vi "Launch VI Tester.vi"(8 "error in (no error)":errorcluster, 11 "application reference":refnum<vi>) -> (0 "error out":errorcluster, 2 "Opened UI?":bool, 3 "VI Tester Ref":refnum<vi>)   [LabVIEW 2011, in "VI Tester Project API.lvlib"]
uses:
  VI Tester Project API.lvlib
panel:
  out "Status":string
  out "Version":string
  # "© 2007 - 2014 JKI. All Rights Reserved."
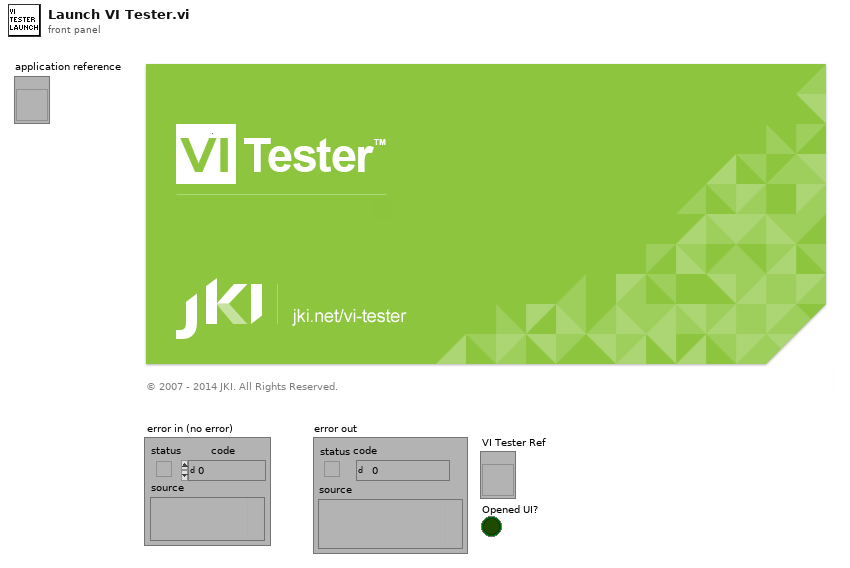
[diagram p1: front panel]
types:
  T1 = enum32{"Bad", "Idle", "Run top level", "Running"}
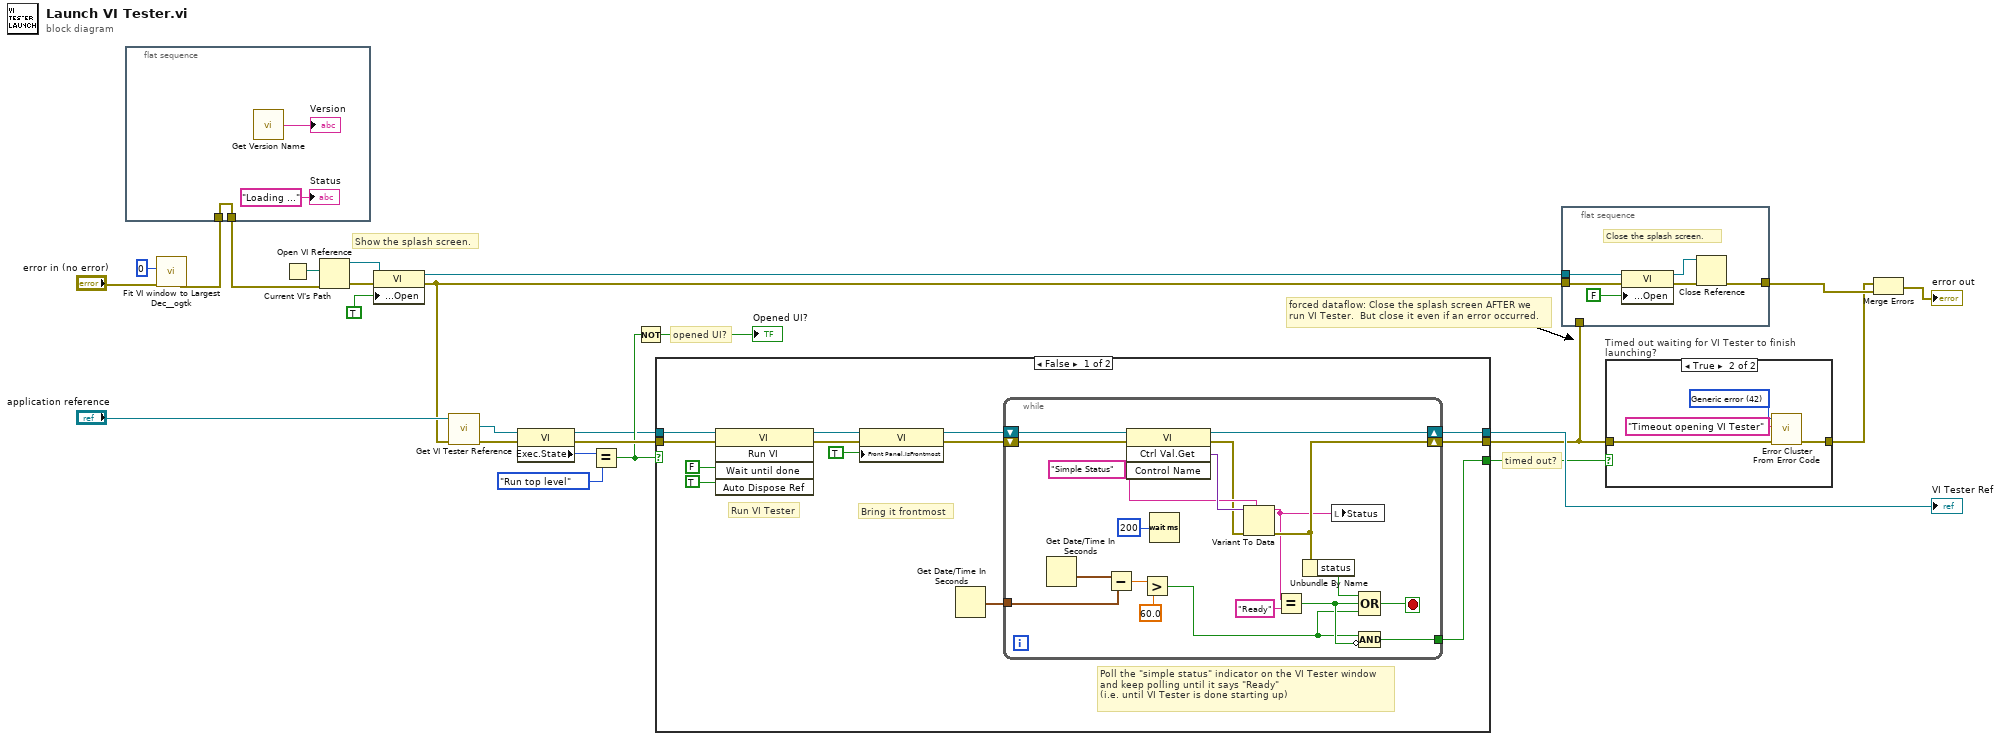
[diagram p0: block diagram]
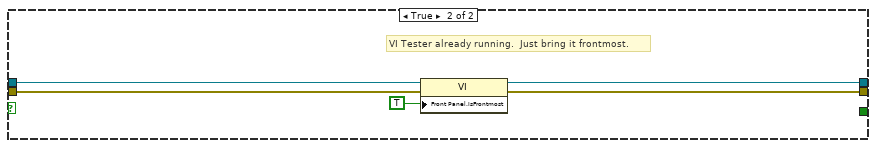
[diagram p3: hidden frame]
diagram:
  # "timed out?"
  # "forced dataflow: Close the splash screen AFTER we\nrun VI Tester.  But close it even if an error occurred."
  # "Show the splash screen."
  # "opened UI?"
  n1 = flat-sequence {
    tunnel: [w27] -> w1
    tunnel: w2 -> [w27]
    frame #0 {
      n2 = call "Get Version Name.vi"() -> ("Version Name"=→"Version":string)
      "Status" <- "Loading ..." ("Status")
    }
  }
  n3 = call <userlib>:"Fit VI window to Largest Dec__ogtk.vi"("error in (no error)"="error in (no error)", "border spacing (2 px)"=0) -> ("error out"=w2:errorcluster)  [unwired: 4 in, 1 out]
  n4 = Current VI's Path() -> (path=w20:path)
  n5 = Open VI Reference(vi path=w20, error in (no error)=w1) -> (vi reference=w22:refnum<vi>, error out=w21:errorcluster)  [unwired: 4 in]
  n6 = property class="VI"(reference=w22, error in=w21, "Front Panel Window:Open"=TRUE) -> (reference out=w17:refnum<vi>, error out=w4:errorcluster)
  n7 = call "Get VI Tester Reference.vi"("error in"=w4, "application reference (This Application)"="application reference") -> ("error out"=w14:errorcluster, "vi reference"=w5:refnum<vi>)  [unwired: 8 in]
  n8 = property class="VI"(reference=w5, error in=w14) -> (reference out=w9:refnum<vi>, error out=w23:errorcluster, "Exec.State"=w25:T1)
  n9 = Equal?(x=w25, y=T1."Run top level") -> (x = y?=w10:bool)
  n10 = Not(x=w10) -> (.not. x?=→"Opened UI?":bool)
  n11 = case shown="False" w10 {
    tunnel: w23 -> [w41 w64]
    tunnel: w9 -> [w38 w65]
    tunnel: [w30 w61] -> w3
    tunnel: [w32 w62] -> w7
    tunnel: [w29 _] -> w6
    frame False {
      # "Poll the \"simple status\" indicator on the VI Tester window\nand keep polling until it says \"Ready\"\n(i.e. until VI Tester is done starting up)"
      # "Bring it frontmost"
      # "Run VI Tester"
      n12 = invoke class="VI" method="Run VI"(reference=w38, error in=w41, "Wait until done"=FALSE ("Wait Until Done"), "Auto Dispose Ref"=TRUE ("Auto Dispose Reference")) -> (reference out=w36:refnum<vi>, error out=w35:errorcluster)  [unwired: 1 in, 3 out]
      n13 = property class="VI"(reference=w36, error in=w35, "Front Panel.IsFrontmost"=TRUE ("Front Panel Window:Is Frontmost")) -> (reference out=w33:refnum<vi>, error out=w31:errorcluster)
      n14 = Get Date/Time In Seconds() -> (seconds since 1Jan1904=w34:timestamp)
      n15 = while {
        shift-right: [w53] -> w30
        shift-left: w31 -> [w49]
        shift-right: [w58] -> w32
        shift-left: w33 -> [w50]
        tunnel: w34 -> [w43]
        tunnel: [w45] -> w29
        stop <- w48 stop-if-true
        w59 = "Simple Status" ("Control Name")
        n16 = Get Date/Time In Seconds() -> (seconds since 1Jan1904=w56:timestamp)
        n17 = Subtract(x=w56, y=w43) -> (x-y=w55:dbl)
        n18 = invoke class="VI" method="Ctrl Val.Get"(reference=w50, error in=w49, "Control Name"=w59) -> (reference out=w58:refnum<vi>, error out=w57:errorcluster, "Get Control Value Variant"=w60:variant)  [unwired: 1 in, 1 out]
        n19 = Greater?(x=w55, y=60.0) -> (0:w46:bool)
        n20 = Wait (ms)(milliseconds to wait=u32 200) -> ()  [unwired: 1 out]
        n21 = Variant To Data(error in=w57, type=w59, Variant=w60) -> (data=w42:string, error out=w53:errorcluster)
        n22 = Equal?(x=w42, y="Ready") -> (x = y?=w47:bool)
        n23 = Unbundle By Name(w53) -> ("status"=w52:bool)
        n24 = local write "Status"(w42) -> ()
        n25 = Compound Arithmetic op=OR(w52, w47, w46) -> (w48:bool)
        n26 = Compound Arithmetic op=AND(w46, invert w47) -> (w45:bool)
      }
    }
    frame True {
      # "VI Tester already running.  Just bring it frontmost."
      n27 = property class="VI"(reference=w65, error in=w64, "Front Panel.IsFrontmost"=TRUE ("Front Panel Window:Is Frontmost")) -> (reference out=w62:refnum<vi>, error out=w61:errorcluster)
    }
  }
  "VI Tester Ref" <- w7
  n28 = flat-sequence {
    tunnel: w17 -> [w69]
    tunnel: [w67] -> w13
    tunnel: w4 -> [w66]
    tunnel: w3 -> [_]
    frame #0 {
      # "Close the splash screen."
      n29 = property class="VI"(reference=w69, error in=w66, "Front Panel Window:Open"=FALSE) -> (reference out=w70:refnum<vi>, error out=w68:errorcluster)
      n30 = Close Reference(reference=w70, error in (no error)=w68) -> (error out=w67:errorcluster)
    }
  }
  n31 = case "Timed out waiting for VI Tester to finish launching?" shown="True" w6 {
    tunnel: w3 -> [w72 w74]
    tunnel: [w72 w73] -> w8
    frame False {
    }
    frame True {
      w76 = 42 items=["No error", "Argument error", "Memory is full", "Out of zone", "End of file", "File already open", "Generic file I/O error", "File not found", "File permission error", "Disk is full", "Duplicate path", "Too many files open", "System feature not enabled", "Resource file not found", "Cannot add resource", "Resource not found", "Image not found", "Image memory error", "Pen does not exist", "Config type invalid", "Config token not found", "Config parse error", "Config memory error", "Bad external code format", "Bad external code offset", "External code not present", "Null window", "Destroy window error", "Null menu", "Print aborted", "Bad print record", "Print driver error", "Windows error during printing", "Memory error during printing", "Print dialog error", "Generic print error", "Invalid device refnum", "Device not found", "Device parameter error", "Device unit error", "Cannot open device", "Device call aborted", "Generic error", "Cancelled by user", "Object ID too low", "Object ID too high", "Object not in heap", "Unknown heap", "Unknown object (invalid DefProc)", "Unknown object (DefProc not in table)", "Message out of range", "Invalid (null) method", "Unknown message", "Manager call not supported", "Bad address", "Network operation in progress", "Network operation timed out", "Connection is busy", "Network attribute not supported", "Network error", "Address in use", "System out of memory", "Connection aborted", "Connection refused", "Not connected", "Already connected", "Connection closed", "Initialization error (interapplication manager)", "Bad occurrence", "Wait on unbound occurrence handler", "Occurrence queue overflow", "Datalog type conflict", "Unused", "Unrecognized type (interapplication manager)", "Memory corrupt", "Failed to make temporary DLL", "Old CIN version", "Drag socket not found", "Failed to load drop-object", "Failed to register OLE object", "Failed to release OLE object", "Format specifier type mismatch", "Unknown format specifier", "Too few format specifiers", "Too many format specifiers", "Scan failed", "Newer CIN version", "Error converting to variant", "Runtime menu error", "Password tampered", "Variant attribute not found", "Incompatible variant data type", "Event data is not available", "Event Store is not present", "Occurrence is not found", "Event Queue is not created", "Event info is not available", "Refnum passed is NULL", "Error retrieving Class GUID", "Error retrieving CoClass GUID", "Error retrieving TypeLib GUID.", "Bad built application magic bytes.", "Specific driver is different from the specific driver associated with the Logical Name.", "There is no session opened to the class driver.", "Max Error", "MAX - Error with config objects", "MAX - Error loading configuration", "MAX - Group not supported"]
      n32 = call <vilib>:"Error Cluster From Error Code.vi"("error in (no error)"=w74, "error message (\"\")"="Timeout opening VI Tester" ("error message (\"\")"), "error code (0)"=w76) -> ("error out"=w73:errorcluster)  [unwired: 6 in]
    }
  }
  n33 = Merge Errors(w8, w13) -> (→"error out":errorcluster)
